vi "CameraKill.vi"(8 "error in (no error)":errorcluster, 11 "IMAQdx in":refnum<class "IMAQdx_Flea3_Firewire.lvclass">) -> (0 "error out":errorcluster, 3 "IMAQdx out":refnum<class "IMAQdx_Flea3_Firewire.lvclass">)   [LabVIEW 2012, in "IMAQdx_Flea3_Firewire.lvclass"]
uses:
  <userlib>/bias2/classes/IMAQdx_Flea3_Firewire/IMAQdx_Flea3_Firewire.lvclass
  <vilib>/userdefined/High Color/IMAQdx.ctl
  <userlib>/bias2/classes/IMAQdx_Flea3_Firewire/IMAQdx_Flea3_Firewire.lvclass/IMAQdx_Flea3_Firewire.ctl
  <vilib>/vision/driver/NI_Vision_Acquisition_Software.lvlib
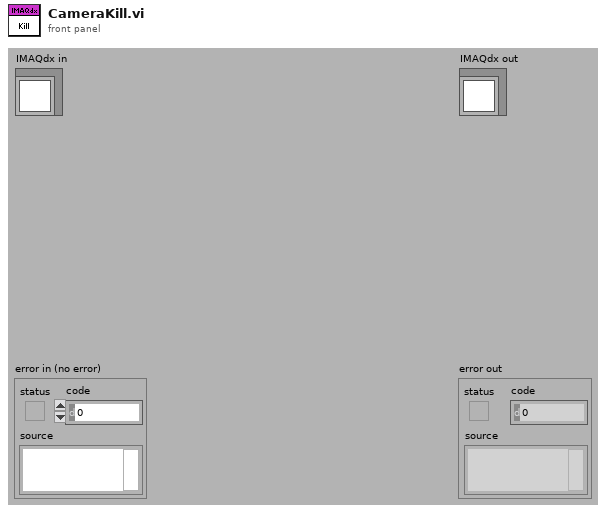
[diagram p1: front panel]
types:
  T1 = typedef "IMAQdx.ctl" = refnum<k21>
  T2 = typedef "IMAQ Image.ctl" = refnum<image>
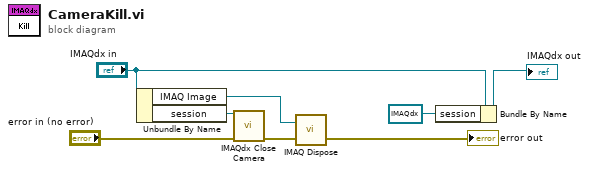
[diagram p0: block diagram]
diagram:
  n1 = Unbundle By Name("IMAQdx in") -> ("IMAQ Image"=w3:T2, "session"=w8:refnum<k21>)
  n2 = call <vilib>:"IMAQdx Close Camera.vi"("error in"="error in (no error)", "Session In"=w8) -> ("error out"=w2:errorcluster)  [unwired: 9 in]
  n3 = call "IMAQ Dispose"("Image"=w3, "error in (no error)"=w2) -> ("error out"=→"error out":errorcluster)  [unwired: 4 in]
  n4 = Bundle By Name(cluster="IMAQdx in", "session"=T1 refnum) -> (→"IMAQdx out":refnum<class "IMAQdx_Flea3_Firewire.lvclass">)
